vi "On Line Calibration.vi"(0 "error in (no error)":errorcluster, 7 "isSubVI":bool=TRUE, 10 "Session In":T1="cam1", 11 "Dove salvo l'immagine Calib Info":path=path "C:/Users/Dell/Documents/UNIVERSITA'/SistemiDiVisione/LabView/On Line calibration/calib-info.png") -> (3 "Calibration Axis Info":T4={"Origin Pixel"={"X"=44.15415, "Y"=79.22556}, "Angle Relative to Horizontal (deg)"=0.0, "X Axis Pixel"={"X"=0.0, "Y"=0.0}, "Axis Reference"=1} {"X Axis Pixel"."Y" format="%.2f"; "X Axis Pixel"."X" format="%.2f"; "Axis Reference" items=["Direct", "Indirect"]; "Angle Relative to Horizontal (deg)" format="%.2f"; "Origin Pixel"."Y" format="%.2f"; "Origin Pixel"."X" format="%.2f"}, 8 "error out":errorcluster)   [LabVIEW 2020]
uses:
  <vilib>/vision/Calibration.llb/Error Statistics.ctl
  <vilib>/userdefined/High Color/IMAQdx.ctl
panel:
  out "Error Map":sgl[][](array[numeric]) format="%.2f"
  out "Error Statistics":T2
  in  "Grid Descriptor 2":cluster{"X Step":sgl, "Y Step":sgl, "Unit":T3}={"X Step"=10.0, "Y Step"=10.0, "Unit"=enum."Millimeter"}
  out "Preprocessed image":T5(plugin-control)
  out "Input Calibration Grid":T5(plugin-control)
  in  "Stop Acquisizione":bool
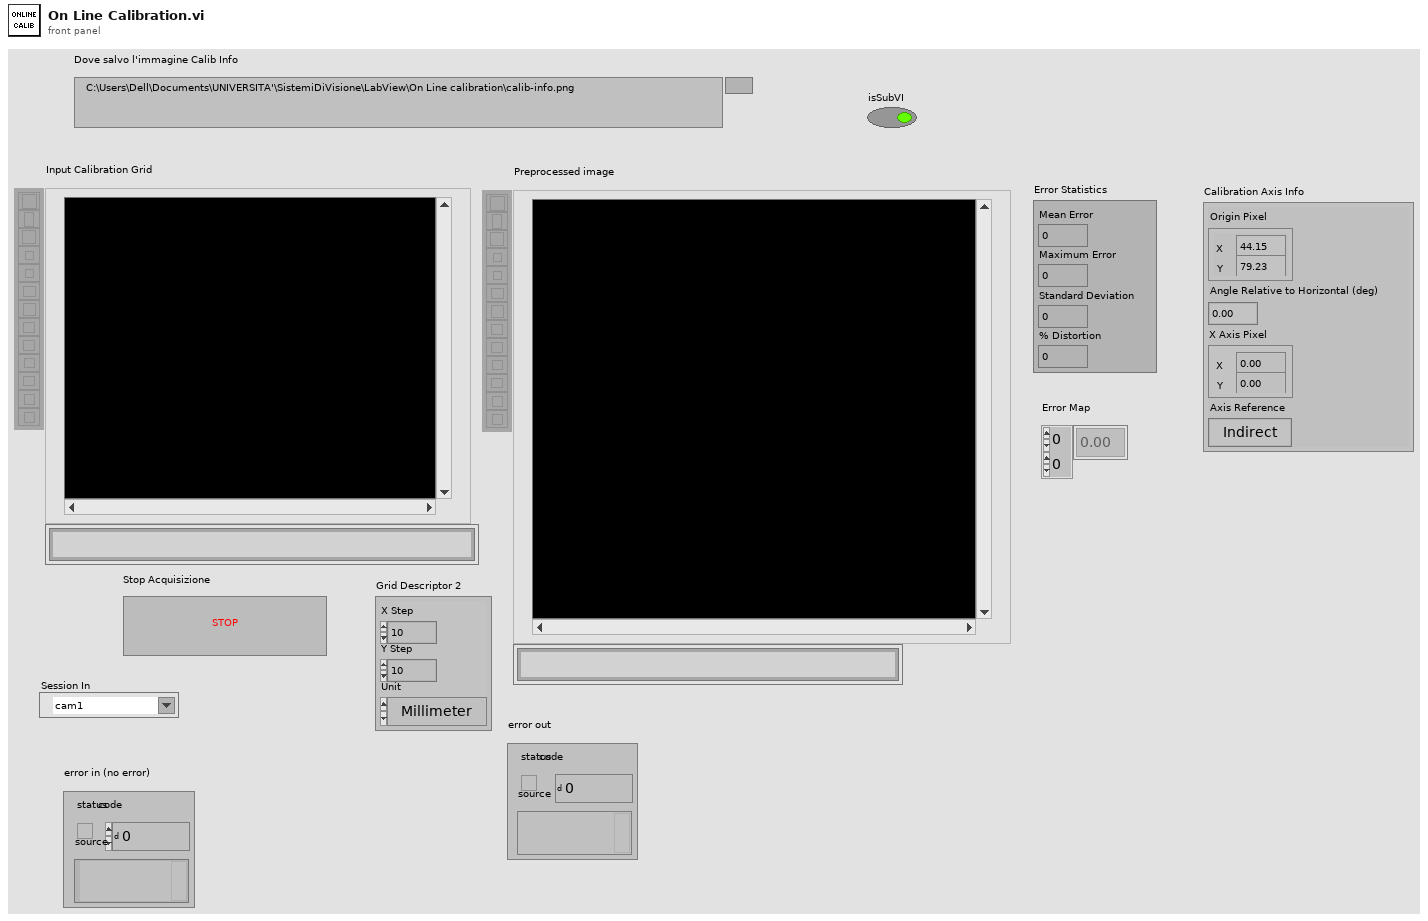
[diagram p1: front panel]
types:
  T1 = typedef "IMAQdx.ctl" = refnum<k21>
  T2 = typedef "Error Statistics.ctl" = cluster{"Mean Error":dbl, "Maximum Error":dbl, "Standard Deviation":dbl, "% Distortion":dbl}
  T3 = typedef "Image Unit" = enum32{"Undefined", "Angström", "Micrometer", "Millimeter", "Centimeter", "Meter", "Kilometer", "Microinch", "Inch", "Feet", "Nautical miles", "Standard miles", "Steps"}
  T4 = cluster{"Origin Pixel":cluster{"X":sgl, "Y":sgl}, "Angle Relative to Horizontal (deg)":sgl, "X Axis Pixel":cluster{"X":sgl, "Y":sgl}, "Axis Reference":u32}
  T5 = typedef "IMAQ Image.ctl" = refnum<image>
  T6 = typedef "Calibration Reference Points.ctl" = cluster{"Pixel Coordinates":cluster{"X":dbl, "Y":dbl}[], "Real World Coordinates":cluster{"X":dbl, "Y":dbl}[], "Unit":T3, "Image Size":cluster{"X":u32, "Y":u32}}
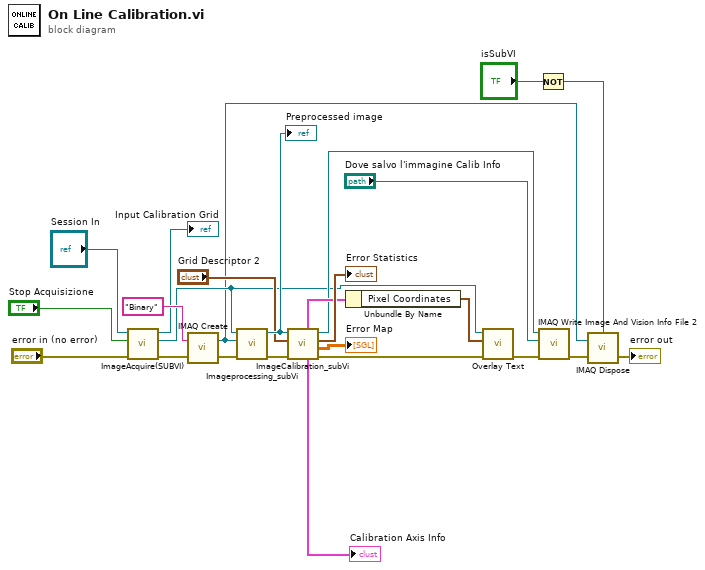
[diagram p0: block diagram]
diagram:
  n1 = call "ImageAcquire(SUBVI).vi"("error in (no error)"="error in (no error)", "Stop Acquisizione"="Stop Acquisizione", "Refnum in"="Session In") -> ("error out"=w7:errorcluster, "Image Dst Out"=w11:T5, "Refnum out"=→"Input Calibration Grid":T5)  [unwired: 6 in]
  n2 = call "IMAQ Create"("Image Name"="Binary", "error in (no error)"=w7) -> ("New Image"=w4:T5, "error out"=w6:errorcluster)  [unwired: 3 in]
  n3 = call "Imageprocessing_subVi.vi"("error in (no error)"=w6, "Binary Img"=w4, "Image In"=w11) -> ("error out"=w23:errorcluster, "Image Dst Out"=w21:T5)  [unwired: 7 in]
  "Preprocessed image" <- w21
  n4 = call "ImageCalibration_subVi.vi"("error in (no error)"=w23, "Grid Descriptor"="Grid Descriptor 2", "Preprocedded Img In"=w21) -> ("error out"=w13:errorcluster, "Error Map"=→"Error Map":sgl[][], "Error Statistics"=→"Error Statistics":T2, "Calibration Template Image (duplicate)"=w15:T5, "Calibration Axis Info"=→"Calibration Axis Info":T4, "Reference Points"=w17:T6)  [unwired: 3 in]
  n5 = Unbundle By Name(w17) -> ("Pixel Coordinates"=w10:cluster{"X":dbl, "Y":dbl}[])
  n6 = call "Overlay Text.vi"("error in (no error)"=w13, "Pixel Coordinates"=w10, "Refnum in"=w11) -> ("error out"=w12:errorcluster)  [unwired: 8 in]
  n7 = Not(x="isSubVI") -> (.not. x?=w1:bool)
  n8 = call "IMAQ Write Image And Vision Info File 2"("error in (no error)"=w12, "File Path"="Dove salvo l'immagine Calib Info", "Image"=w15) -> ("error out"=w3:errorcluster)  [unwired: 7 in, 1 out]
  n9 = call "IMAQ Dispose"("All Images? (No)"=w1, "Image"=w4, "error in (no error)"=w3) -> ("error out"=→"error out":errorcluster)  [unwired: 3 in]
